vi "HEWH Panel Collect Data for Specific Time.vi"(8 "error in (no error)":errorcluster) -> (0 "error out":errorcluster, 1 "Back Button":bool, 2 "Elapsed Time Output":T2 format="%<%H:%M:%S>t", 3 "Continuous Data Collection Output":bool)   [LabVIEW 2019]
uses:
  Utility/Custom Pallet Controls/Custom Pallet Forward.ctl
  Utility/Custom Pallet Controls/Custom Pallet Timer.ctl
  Utility/Custom Pallet Controls/Custom Pallet Reverse.ctl
panel:
  in  "Back Button":T1
  out "Description":string="Data Collection Setup"
  in  "Elapsed Time":T2 format="%<%H:%M:%S>t"
  in  "Specific Time":bool
  in  "Continuous Data Collection":bool
  in  "File Setup OK":T3
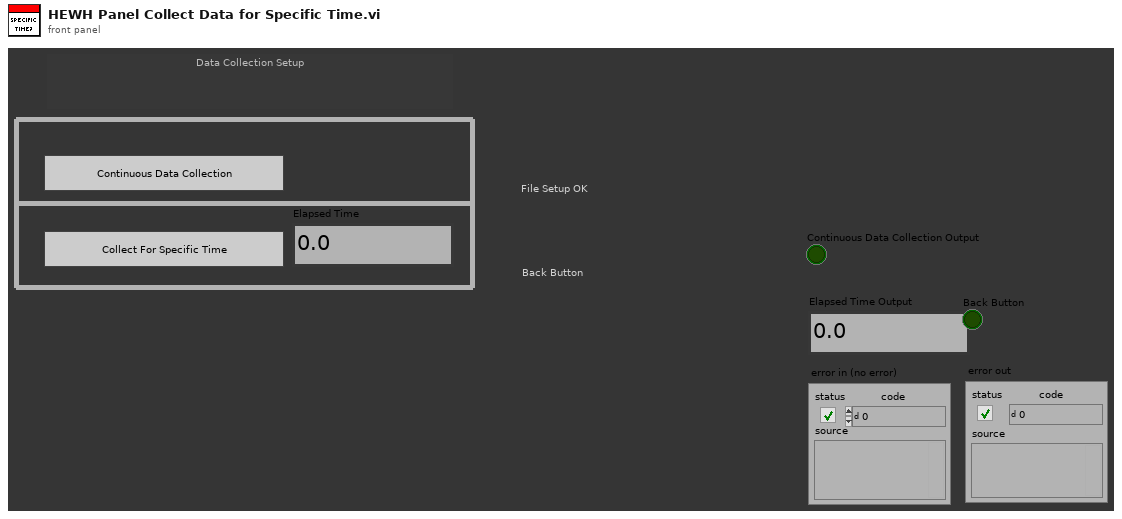
[diagram p1: front panel]
types:
  T1 = typedef "Custom Pallet Reverse.ctl" = bool
  T2 = typedef "Custom Pallet Timer.ctl" = dbl
  T3 = typedef "Custom Pallet Forward.ctl" = bool
  T4 = enum32{"invalid app kind", "Development System", "Run Time System", "Student Edition", "Embedded LabVIEW", "Evaluation", "Custom"}
  T5 = enum32{"Invalid", "Standard", "Closed", "Hidden", "Minimized", "Maximized"}
  T6 = cluster{"Core":cluster{"Current VI Reference":refnum<vi>, "Close Panel on Exit?":bool}, "Elapsed Time":T2, "Continuous Data Collection":bool}
  T7 = cluster{"Current VI Reference":refnum<vi>, "Close Panel on Exit?":bool}
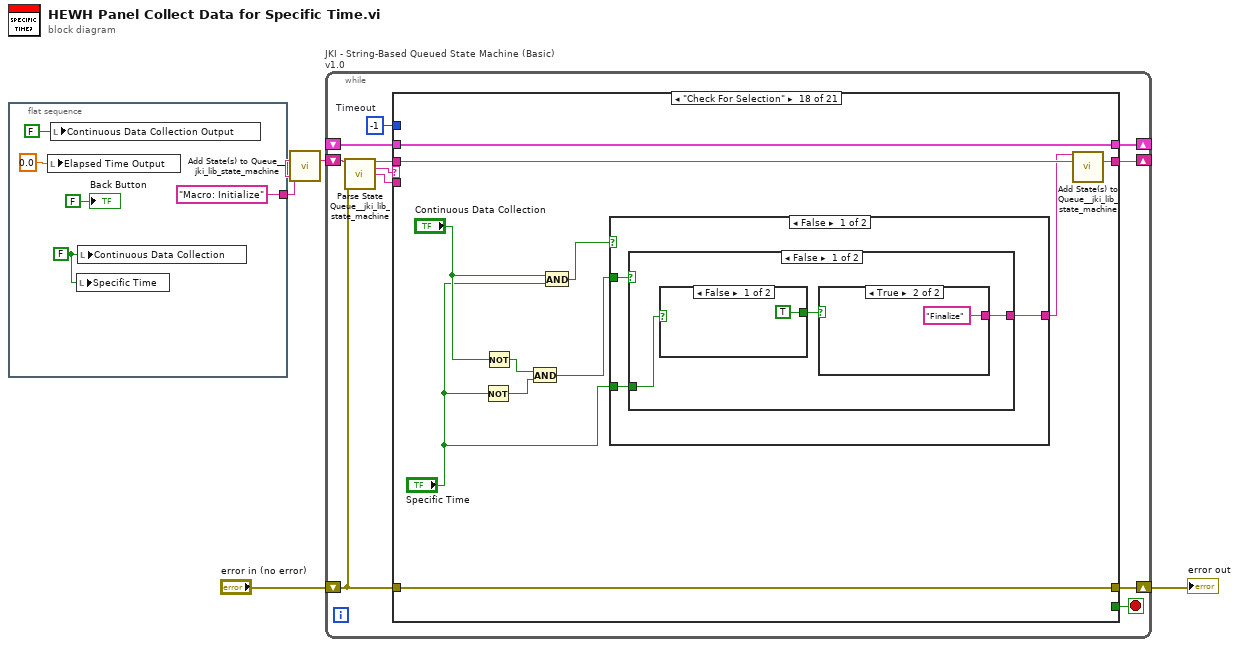
[diagram p0: block diagram]
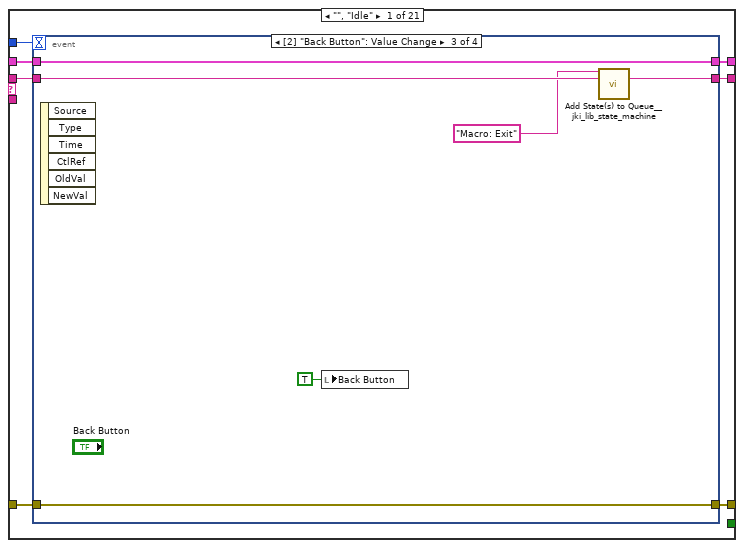
[diagram p2: hidden frame]
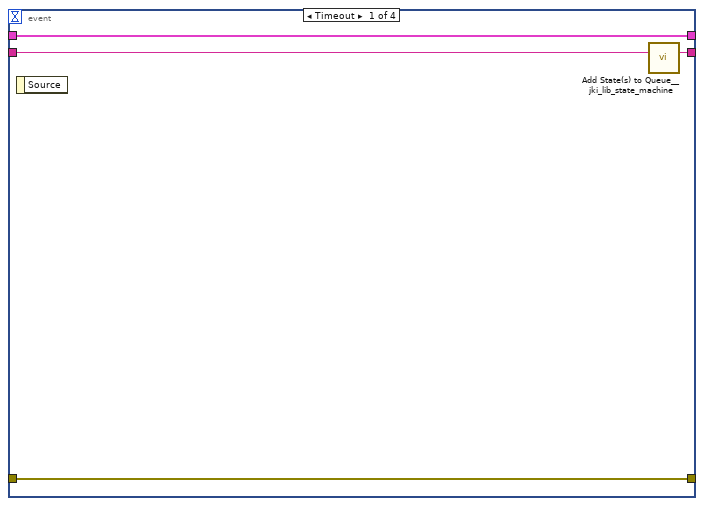
[diagram p3: hidden frame]
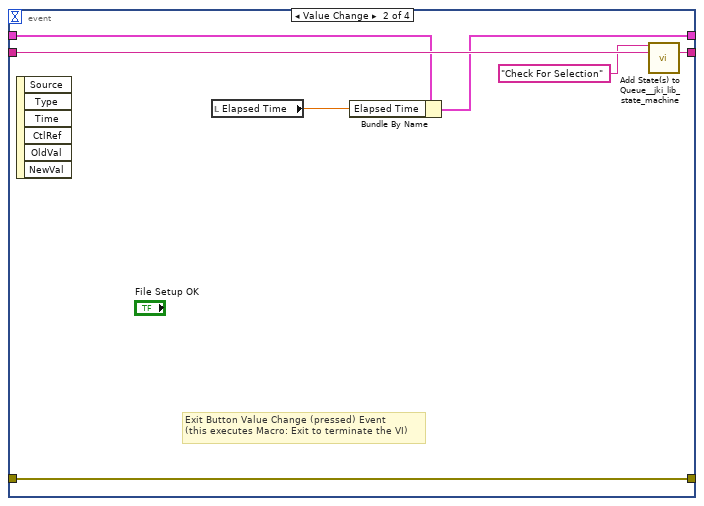
[diagram p4: hidden frame]
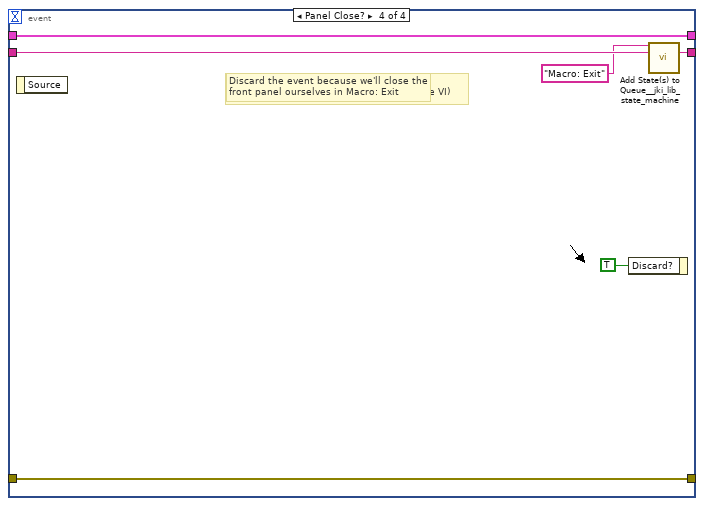
[diagram p5: hidden frame]
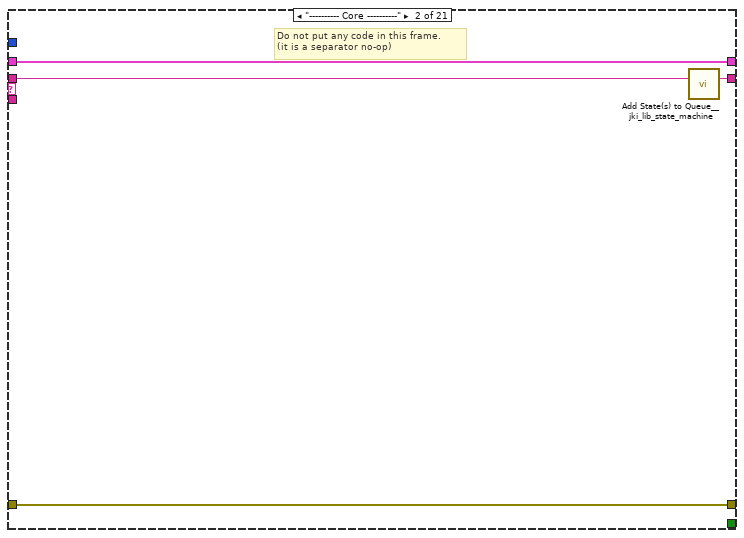
[diagram p6: hidden frame]
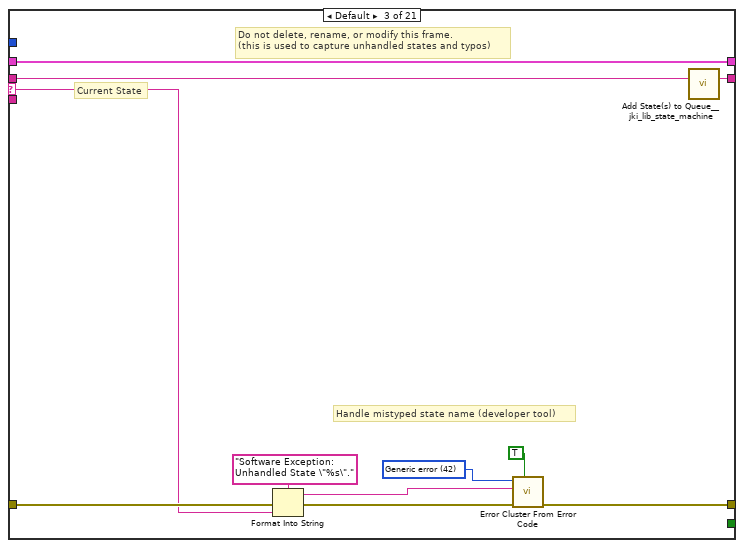
[diagram p7: hidden frame]
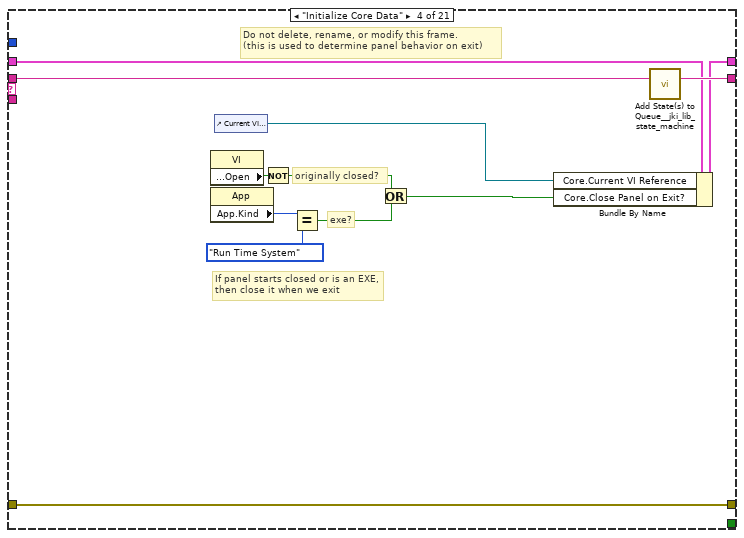
[diagram p8: hidden frame]
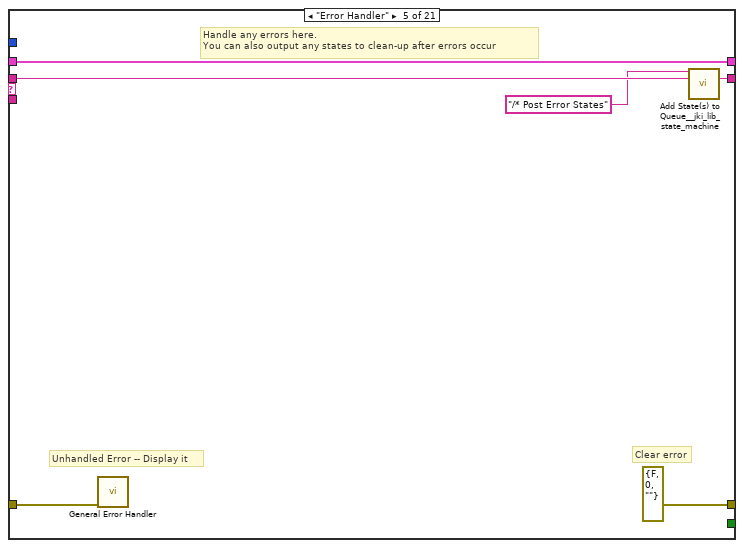
[diagram p9: hidden frame]
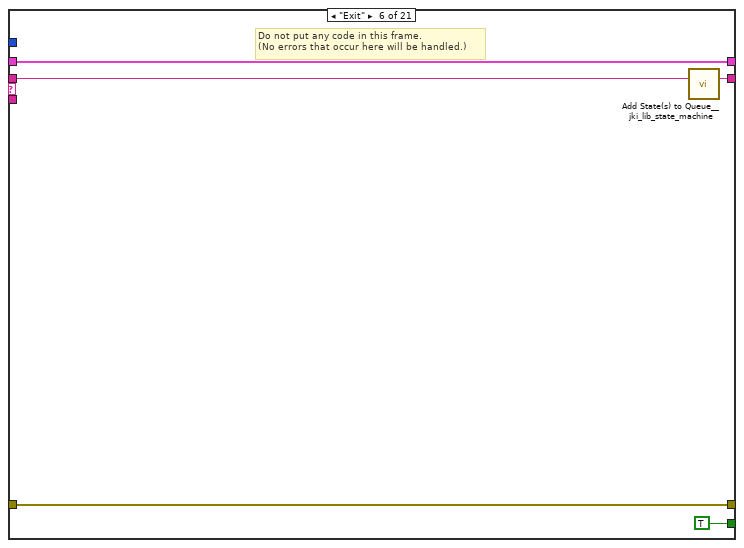
[diagram p10: hidden frame]
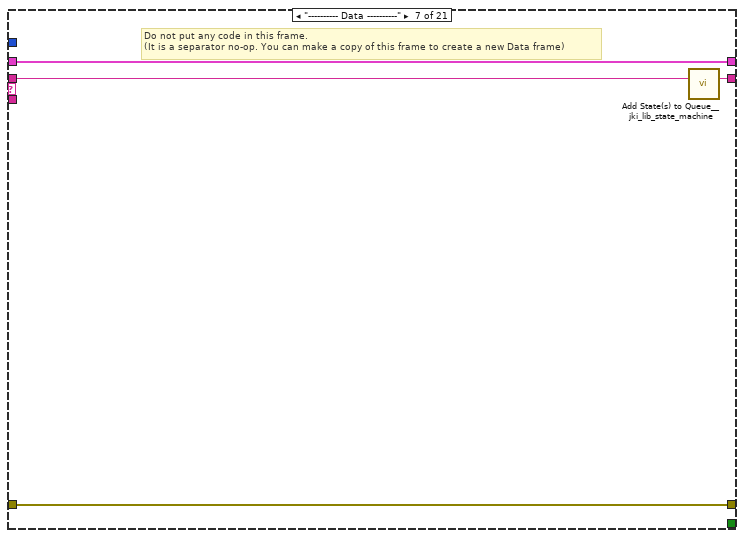
[diagram p11: hidden frame]
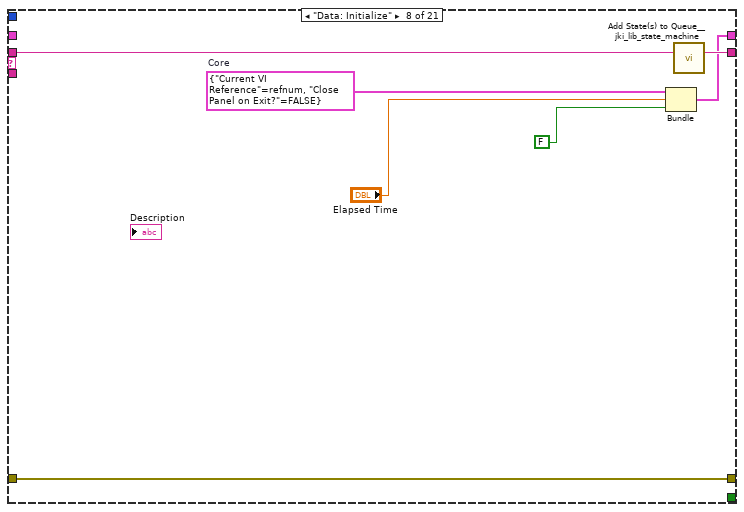
[diagram p12: hidden frame]
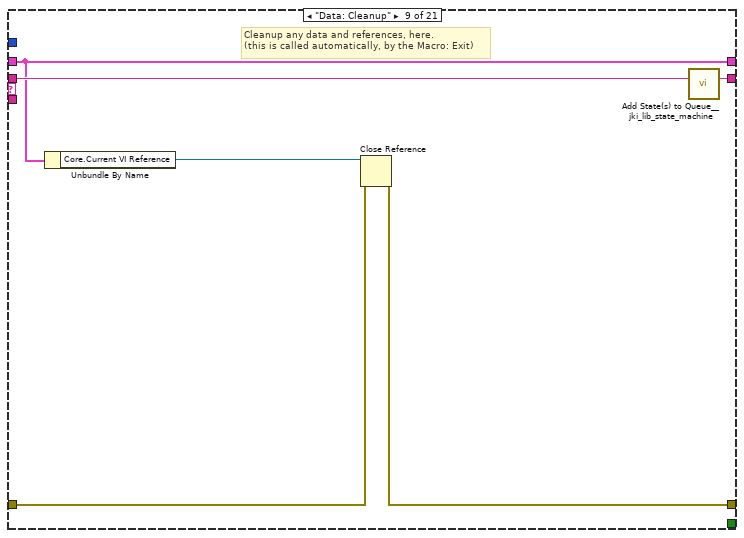
[diagram p13: hidden frame]
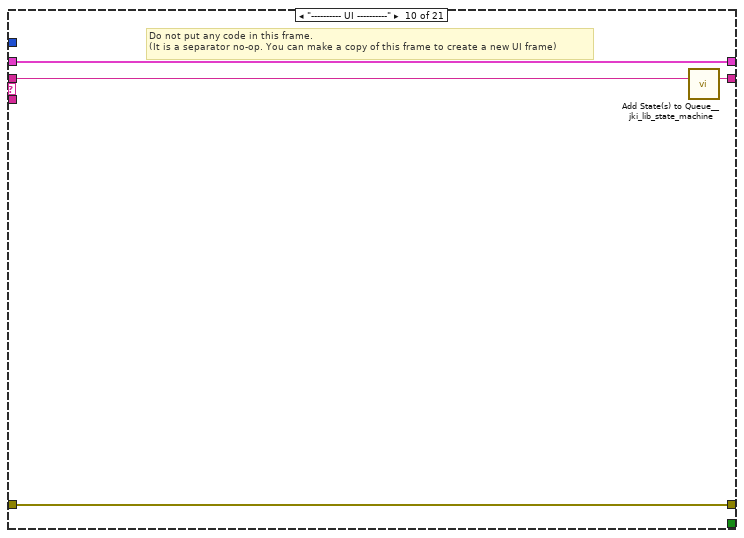
[diagram p14: hidden frame]
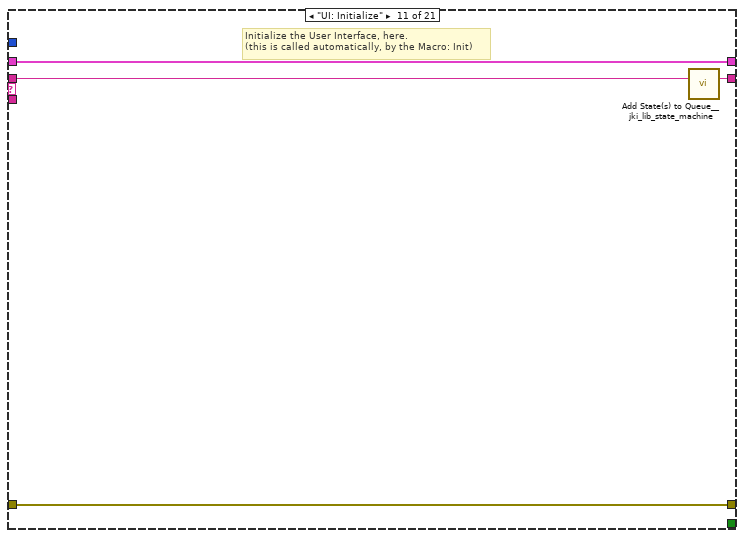
[diagram p15: hidden frame]
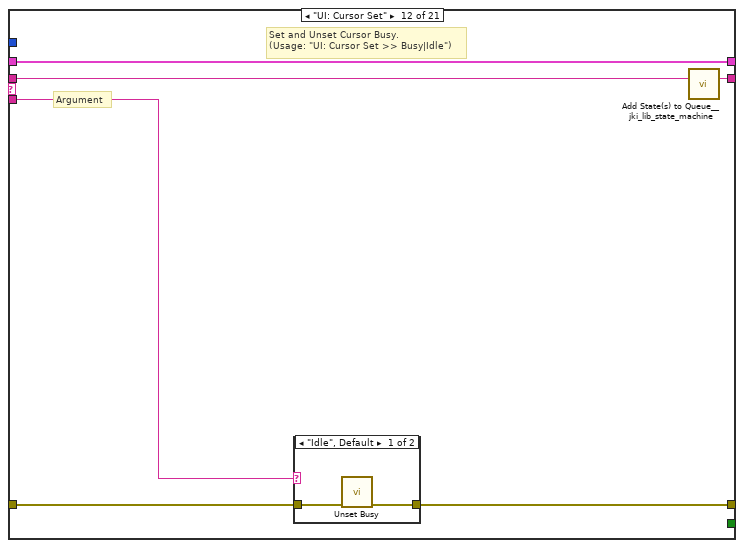
[diagram p16: hidden frame]
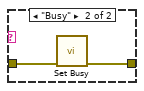
[diagram p17: hidden frame]
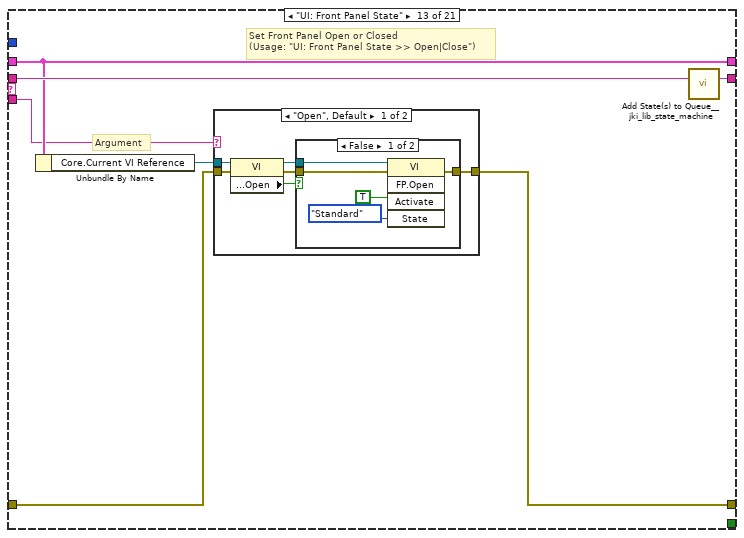
[diagram p18: hidden frame]
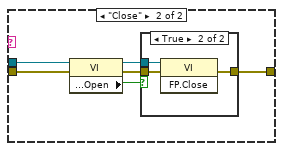
[diagram p20: hidden frame]
diagram:
  n1 = flat-sequence {
    tunnel: ["Macro: Initialize"] -> w3
    frame #0 {
      w5 = FALSE ("Continuous Data Collection")
      n2 = local write "Elapsed Time Output"(T2 0.0 ("Elapsed Time Output")) -> ()
      n3 = local write "Continuous Data Collection Output"(FALSE ("Continuous Data Collection Output")) -> ()
      n4 = local write "Specific Time"(w5) -> ()
      n5 = local write "Continuous Data Collection"(w5) -> ()
      "Back Button" <- FALSE ("Back Button")
    }
  }
  n6 = call <vilib>:"Add State(s) to Queue__jki_lib_state_machine.vi"("State(s) in (\"\")"=w3) -> ("States Out"=w4:string)  [unwired: 14 in]
  n7 = while "JKI - String-Based Queued State Machine (Basic) v1.0" {
    shift-right: [w13] -> _
    shift-left: _ -> [w12]
    shift-right: [w16] -> w2
    shift-left: "error in (no error)" -> [w10]
    shift-right: [w15] -> _
    shift-left: w4 -> [w17]
    stop <- w14 stop-if-true
    w11 = -1  # Timeout
    n8 = call <vilib>:"Parse State Queue__jki_lib_state_machine.vi"("State Queue"=w17, "Error In (no error)"=w10) -> ("Remaining States"=w19:string, "Current State"=w20:string, "Arguments"=w18:string)  [unwired: 11 in]
    n9 = case shown="\"Check For Selection\"" w20 {
      selector: w20 -> [_ _ w55 _ _ _ _ _ _ _ _ _ _ _ _ _ _ _ _ _ _]
      tunnel: w19 -> [w27 w54 w59 w77 w83 w88 w92 w99 w105 w109 w113 w119 w130 w156 w161 w171 w175 w186 w209 w221 w228]
      tunnel: w18 -> [_ _ _ _ _ _ _ _ _ _ _ w114 w124 _ _ _ _ _ _ _ _]
      tunnel: w12 -> [w25 w51 w57 w68 w80 w86 w89 _ w100 w106 w111 w117 w126 w153 w158 w168 w172 w183 w205 w218 w225]
      tunnel: [w24 w52 w61 w74 errorcluster {"status"=FALSE, "code"=0, "source"=""} ("error out") w85 w90 w96 w101 w107 w110 w115 w127 w154 w159 w169 w173 w184 w207 w219 w226] -> w16
      tunnel: w10 -> [w23 w52 w60 w74 w79 w85 w90 w96 w102 w107 w110 w116 w128 w154 w159 w169 w173 w184 w207 w219 w226]
      tunnel: [w26 w53 w58 w76 w82 w87 w91 w98 w104 w108 w112 w118 w129 w155 w160 w170 w174 w185 w208 w220 w227] -> w15
      tunnel: [_ _ _ _ _ TRUE _ _ _ _ _ _ _ _ _ _ _ _ _ _ _] -> w14
      tunnel: [w22 w51 w57 w75 w80 w86 w89 w97 w100 w106 w111 w117 w126 w153 w158 w168 w172 w183 w204 w218 w225] -> w13
      tunnel: w11 -> [w21 _ _ _ _ _ _ _ _ _ _ _ _ _ _ _ _ _ _ _ _]
      frame "", "Idle" {
        n10 = event shown="[2] \"Back Button\": Value Change" {
          selector: _ -> [_ _ _ _]
          dyn-events: _ -> [_ _ _ _]
          timeout: w21 -> [_ _ _ _]
          tunnel: w27 -> [w31 w38 w41 w50]
          tunnel: [w30 w37 w40 w49] -> w26
          tunnel: w25 -> [w28 w34 w43 w47]
          tunnel: [w29 w36 w44 w48] -> w24
          tunnel: w23 -> [w29 w36 w44 w48]
          tunnel: [w28 w33 w43 w47] -> w22
          event Timeout {
            n11 = event-data() -> ()  [unwired: 1 in, 1 out]
            n12 = call <vilib>:"Add State(s) to Queue__jki_lib_state_machine.vi"("State(s) in (\"\")"=w31) -> ("States Out"=w30:string)  [unwired: 14 in]
          }
          event Value Change {
            # "Exit Button Value Change (pressed) Event\n(this executes Macro: Exit to terminate the VI)"
            n13 = event-data() -> ()  [unwired: 1 in, 6 out]
            n14 = local read "Elapsed Time"() -> (w32:T2)
            n15 = Bundle By Name(cluster=w34, "Elapsed Time"=w32) -> (w33:T6)
            n16 = call <vilib>:"Add State(s) to Queue__jki_lib_state_machine.vi"("State(s) in Front (\"\")"="Check For Selection", "State(s) in (\"\")"=w38) -> ("States Out"=w37:string)  [unwired: 13 in]
          }
          event Value Change {
            n17 = event-data() -> ()  [unwired: 1 in, 6 out]
            n18 = local write "Back Button"(TRUE ("Back Button")) -> ()
            n19 = call <vilib>:"Add State(s) to Queue__jki_lib_state_machine.vi"("State(s) in Front (\"\")"="Macro: Exit" ("State(s) in Front (\"\")"), "State(s) in (\"\")"=w41) -> ("States Out"=w40:string)  [unwired: 13 in]
          }
          event Panel Close? {
            # "Discard the event because we'll close the front panel ourselves in Macro: Exit"
            # "Close Panel button (pressed) Event\n(this executes Macro: Exit to terminate the VI)"
            n20 = event-data() -> ()  [unwired: 1 in, 1 out]
            n21 = event-data("Discard?"=TRUE) -> ()  [unwired: 1 in, 1 out]
            n22 = call <vilib>:"Add State(s) to Queue__jki_lib_state_machine.vi"("State(s) in Front (\"\")"="Macro: Exit", "State(s) in (\"\")"=w50) -> ("States Out"=w49:string)  [unwired: 13 in]
          }
        }
      }
      frame "---------- Core ----------" {
        # "Do not put any code in this frame.\n(it is a separator no-op)"
        n23 = call <vilib>:"Add State(s) to Queue__jki_lib_state_machine.vi"("State(s) in (\"\")"=w54) -> ("States Out"=w53:string)  [unwired: 14 in]
      }
      frame Default {
        w64 = 42 items=["No error", "Argument error", "Memory is full", "Out of zone", "End of file", "File already open", "Generic file I/O error", "File not found", "File permission error", "Disk is full", "Duplicate path", "Too many files open", "System feature not enabled", "Resource file not found", "Cannot add resource", "Resource not found", "Image not found", "Image memory error", "Pen does not exist", "Config type invalid", "Config token not found", "Config parse error", "Config memory error", "Bad external code format", "Bad external code offset", "External code not present", "Null window", "Destroy window error", "Null menu", "Print aborted", "Bad print record", "Print driver error", "Windows error during printing", "Memory error during printing", "Print dialog error", "Generic print error", "Invalid device refnum", "Device not found", "Device parameter error", "Device unit error", "Cannot open device", "Device call aborted", "Generic error", "Cancelled by user", "Object ID too low", "Object ID too high", "Object not in heap", "Unknown heap", "Unknown object (invalid DefProc)", "Unknown object (DefProc not in table)", "Message out of range", "Invalid (null) method", "Unknown message", "Manager call not supported", "Bad address", "Network operation in progress", "Network operation timed out", "Connection is busy", "Network attribute not supported", "Network error", "Address in use", "System out of memory", "Connection aborted", "Connection refused", "Not connected", "Already connected", "Connection closed", "Initialization error (interapplication manager)", "Bad occurrence", "Wait on unbound occurrence handler", "Occurrence queue overflow", "Datalog type conflict", "Unused", "Unrecognized type (interapplication manager)", "Memory corrupt", "Failed to make temporary DLL", "Old CIN version", "Drag socket not found", "Failed to load drop-object", "Failed to register OLE object", "Failed to release OLE object", "Format specifier type mismatch", "Unknown format specifier", "Too few format specifiers", "Too many format specifiers", "Scan failed", "Newer CIN version", "Error converting to variant", "Runtime menu error", "Password tampered", "Variant attribute not found", "Incompatible variant data type", "Event data is not available", "Event Store is not present", "Occurrence is not found", "Event Queue is not created", "Event info is not available", "Refnum passed is NULL", "Error retrieving Class GUID", "Error retrieving CoClass GUID", "Error retrieving TypeLib GUID.", "Bad built application magic bytes.", "Specific driver is different from the specific driver associated with the Logical Name.", "There is no session opened to the class driver.", "Max Error", "MAX - Error with config objects", "MAX - Error loading configuration", "MAX - Group not supported"]
        # "Current State"
        # "Do not delete, rename, or modify this frame.\n(this is used to capture unhandled states and typos)"
        # "Handle mistyped state name (developer tool)"
        n24 = Format Into String(format string="Software Exception: Unhandled State \"%s\"." ("message"), error in=w60, w55) -> (resulting string=w63:string, error out=w62:errorcluster)  [unwired: 1 in]
        n25 = call <vilib>:"Error Cluster From Error Code.vi"("show call chain? (False)"=TRUE, "error in (no error)"=w62, "error message (\"\")"=w63, "error code (0)"=w64) -> ("error out"=w61:errorcluster)  [unwired: 5 in]
        n26 = call <vilib>:"Add State(s) to Queue__jki_lib_state_machine.vi"("State(s) in (\"\")"=w59) -> ("States Out"=w58:string)  [unwired: 14 in]
      }
      frame "Initialize Core Data" {
        # "Do not delete, rename, or modify this frame.\n(this is used to determine panel behavior on exit)"
        # "originally closed?"
        # "exe?"
        # "If panel starts closed or is an EXE, then close it when we exit"
        n27 = property class="VI"() -> ("Front Panel.Open"=w73:bool)  [unwired: 2 in, 2 out]
        n28 = property class="App"() -> ("App.Kind"=w72:T4)  [unwired: 2 in, 2 out]
        n29 = control-ref of="Current VI Reference"() -> (w66:refnum<vi>)
        n30 = Not(x=w73) -> (.not. x?=w70:bool)
        n31 = Equal?(x=w72, y=T4."Run Time System" ("Application:Kind")) -> (x = y?=w69:bool)
        n32 = Or(x=w70, y=w69) -> (x .or. y?=w67:bool)
        n33 = Bundle By Name(cluster=w68, "Core.Current VI Reference"=w66, "Core.Close Panel on Exit?"=w67) -> (w75:T6)
        n34 = call <vilib>:"Add State(s) to Queue__jki_lib_state_machine.vi"("State(s) in (\"\")"=w77) -> ("States Out"=w76:string)  [unwired: 14 in]
      }
      frame "Error Handler" {
        # "Unhandled Error -- Display it"
        # "Handle any errors here.\nYou can also output any states to clean-up after errors occur"
        # "Clear error"
        n35 = call <vilib>:"General Error Handler.vi"("error in (no error)"=w79) -> ()  [unwired: 10 in, 5 out]
        n36 = call <vilib>:"Add State(s) to Queue__jki_lib_state_machine.vi"("State(s) in Front (\"\")"="/* Post Error States", "State(s) in (\"\")"=w83) -> ("States Out"=w82:string)  [unwired: 13 in]
      }
      frame "Exit" {
        # "Do not put any code in this frame.\n(No errors that occur here will be handled.)"
        n37 = call <vilib>:"Add State(s) to Queue__jki_lib_state_machine.vi"("State(s) in (\"\")"=w88) -> ("States Out"=w87:string)  [unwired: 14 in]
      }
      frame "---------- Data ----------" {
        # "Do not put any code in this frame.\n(It is a separator no-op. You can make a copy of this frame to create a new Data frame)"
        n38 = call <vilib>:"Add State(s) to Queue__jki_lib_state_machine.vi"("State(s) in (\"\")"=w92) -> ("States Out"=w91:string)  [unwired: 14 in]
      }
      frame "Data: Initialize" {
        w95 = T7 {"Current VI Reference"=refnum, "Close Panel on Exit?"=FALSE}  # Core
        n39 = Bundle("Core"=w95, "Elapsed Time"="Elapsed Time", "Continuous Data Collection"=FALSE) -> (w97:T6)  [unwired: 1 in]
        n40 = call <vilib>:"Add State(s) to Queue__jki_lib_state_machine.vi"("State(s) in (\"\")"=w99) -> ("States Out"=w98:string)  [unwired: 14 in]
      }
      frame "Data: Cleanup" {
        # "Cleanup any data and references, here.\n(this is called automatically, by the Macro: Exit)"
        n41 = Unbundle By Name(w100) -> ("Core.Current VI Reference"=w103:refnum<vi>)
        n42 = Close Reference(reference=w103, error in (no error)=w102) -> (error out=w101:errorcluster)
        n43 = call <vilib>:"Add State(s) to Queue__jki_lib_state_machine.vi"("State(s) in (\"\")"=w105) -> ("States Out"=w104:string)  [unwired: 14 in]
      }
      frame "---------- UI ----------" {
        # "Do not put any code in this frame.\n(It is a separator no-op. You can make a copy of this frame to create a new UI frame)"
        n44 = call <vilib>:"Add State(s) to Queue__jki_lib_state_machine.vi"("State(s) in (\"\")"=w109) -> ("States Out"=w108:string)  [unwired: 14 in]
      }
      frame "UI: Initialize" {
        # "Initialize the User Interface, here.\n(this is called automatically, by the Macro: Init)"
        n45 = call <vilib>:"Add State(s) to Queue__jki_lib_state_machine.vi"("State(s) in (\"\")"=w113) -> ("States Out"=w112:string)  [unwired: 14 in]
      }
      frame "UI: Cursor Set" {
        # "Argument"
        # "Set and Unset Cursor Busy.\n(Usage: \"UI: Cursor Set >> Busy|Idle\")"
        n46 = case shown="\"Idle\", Default" w114 {
          tunnel: w116 -> [w121 w123]
          tunnel: [w120 w122] -> w115
          frame "Idle", Default {
            n47 = call <vilib>:"Unset Busy.vi"("error in (no error)"=w121) -> ("error out"=w120:errorcluster)  [unwired: 10 in]
          }
          frame "Busy" {
            n48 = call <vilib>:"Set Busy.vi"("error in (no error)"=w123) -> ("error out"=w122:errorcluster)  [unwired: 9 in, 1 out]
          }
        }
        n49 = call <vilib>:"Add State(s) to Queue__jki_lib_state_machine.vi"("State(s) in (\"\")"=w119) -> ("States Out"=w118:string)  [unwired: 14 in]
      }
      frame "UI: Front Panel State" {
        # "Argument"
        # "Set Front Panel Open or Closed\n(Usage: \"UI: Front Panel State >> Open|Close\")"
        n50 = Unbundle By Name(w126) -> ("Core.Current VI Reference"=w125:refnum<vi>)
        n51 = case shown="\"Open\", Default" w124 {
          tunnel: w128 -> [w134 w147]
          tunnel: [w136 w148] -> w127
          tunnel: w125 -> [w135 w145]
          frame "Open", Default {
            n52 = property class="VI"(reference=w135, error in=w134) -> (reference out=w132:refnum<vi>, error out=w133:errorcluster, "Front Panel.Open"=w131:bool)
            n53 = case shown="False" w131 {
              tunnel: [w139 w142] -> w136
              tunnel: w133 -> [w138 w142]
              tunnel: w132 -> [w137 _]
              frame False {
                n54 = invoke class="VI" method="FP.Open"(reference=w137, error in=w138, "Activate"=TRUE, "State"=T5."Standard") -> (error out=w139:errorcluster)  [unwired: 1 in, 4 out]
              }
              frame True {
              }
            }
          }
          frame "Close" {
            n55 = property class="VI"(reference=w145, error in=w147) -> (reference out=w144:refnum<vi>, error out=w146:errorcluster, "Front Panel.Open"=w143:bool)
            n56 = case shown="True" w143 {
              tunnel: [w149 w152] -> w148
              tunnel: w146 -> [w149 w151]
              tunnel: w144 -> [_ w150]
              frame False {
              }
              frame True {
                n57 = invoke class="VI" method="FP.Close"(reference=w150, error in=w151) -> (error out=w152:errorcluster)  [unwired: 1 in, 2 out]
              }
            }
          }
        }
        n58 = call <vilib>:"Add State(s) to Queue__jki_lib_state_machine.vi"("State(s) in (\"\")"=w130) -> ("States Out"=w129:string)  [unwired: 14 in]
      }
      frame "---------- Macro ----------" {
        # "Do not put any code in this frame.\n(It is a separator no-op. You can make a copy of this frame to create a new Macro frame)"
        n59 = call <vilib>:"Add State(s) to Queue__jki_lib_state_machine.vi"("State(s) in (\"\")"=w156) -> ("States Out"=w155:string)  [unwired: 14 in]
      }
      frame "Macro: Initialize" {
        w157 = "Data: Initialize\nInitialize Core Data\nUI: Initialize\nUI: Front Panel State >> Open"  # Data: Initialize Initialize Core Data UI: Initialize UI: Front Panel State >> Open
        # "Initialization Macro\n(This is called once, when the VI starts)"
        n60 = call <vilib>:"Add State(s) to Queue__jki_lib_state_machine.vi"("State(s) in Front (\"\")"=w157, "State(s) in (\"\")"=w161) -> ("States Out"=w160:string)  [unwired: 13 in]
      }
      frame "Macro: Exit" {
        # "Exit Macro\n(This is called once, when the VI exits)"
        n61 = Unbundle By Name(w168) -> ("Core.Close Panel on Exit?"=w167:bool)
        n62 = Select(t="UI: Front Panel State >> Close", s=w167, f="") -> (s? t:f=w164:string)
        n63 = call <vilib>:"Add State(s) to Queue__jki_lib_state_machine.vi"("State(s) in (\"\")"=w164, "State(s) at Back (\"\")"="Data: Cleanup\nExit") -> ("States Out"=w162:string)  [unwired: 13 in]
        n64 = call <vilib>:"Add State(s) to Queue__jki_lib_state_machine.vi"("State(s) in Front (\"\")"=w162, "State(s) in (\"\")"=w171) -> ("States Out"=w170:string)  [unwired: 13 in]
      }
      frame "---------- New Category ----------" {
        # "Template Separator\n(You can make a copy of, or modify, this frame)"
        n65 = call <vilib>:"Add State(s) to Queue__jki_lib_state_machine.vi"("State(s) in (\"\")"=w175) -> ("States Out"=w174:string)  [unwired: 14 in]
      }
      frame "Check For Selection" {
        n66 = Not(x="Specific Time") -> (.not. x?=w178:bool)
        n67 = Not(x="Continuous Data Collection") -> (.not. x?=w179:bool)
        n68 = And(x=w179, y=w178) -> (x .and. y?=w177:bool)
        n69 = And(x="Continuous Data Collection", y="Specific Time") -> (x .and. y?=w182:bool)
        n70 = case shown="False" w182 {
          tunnel: [w188 ""] -> w181
          tunnel: w177 -> [w189 _]
          tunnel: "Specific Time" -> [w187 _]
          frame False {
            n71 = case shown="False" w189 {
              tunnel: [w192 ""] -> w188
              tunnel: w187 -> [w190 _]
              frame False {
                n72 = case shown="False" w190 {
                  tunnel: [TRUE w194] -> w191
                  frame False {
                  }
                  frame True {
                    n73 = local read "Elapsed Time"() -> (w195:T2)
                    n74 = Greater Than 0?(x=w195) -> (x > 0?=w194:bool)
                  }
                }
                n75 = case shown="True" w191 {
                  tunnel: ["" "Finalize"] -> w192
                  frame False {
                    n76 = One Button Dialog(message="Enter A Time") -> ()  [unwired: 1 in, 1 out]
                  }
                  frame True {
                  }
                }
              }
              frame True {
                n77 = One Button Dialog(message="Select An Option") -> ()  [unwired: 1 in, 1 out]
              }
            }
          }
          frame True {
            n78 = One Button Dialog(message="Select Only One Option") -> ()  [unwired: 1 in, 1 out]
          }
        }
        n79 = call <vilib>:"Add State(s) to Queue__jki_lib_state_machine.vi"("State(s) in Front (\"\")"=w181, "State(s) in (\"\")"=w186) -> ("States Out"=w185:string)  [unwired: 13 in]
      }
      frame "Finalize" {
        n80 = local read "Continuous Data Collection"() -> (w206:bool)
        n81 = case shown="True" w206 {
          tunnel: w205 -> [w210 w215]
          tunnel: [w210 w214] -> w204
          tunnel: ["Specific Output" "Cont Output"] -> w203
          frame False {
          }
          frame True {
            n82 = Bundle By Name(cluster=w215, "Continuous Data Collection"=TRUE) -> (w214:T6)
          }
        }
        n83 = call <vilib>:"Add State(s) to Queue__jki_lib_state_machine.vi"("State(s) in Front (\"\")"=w203, "State(s) in (\"\")"=w209) -> ("States Out"=w208:string)  [unwired: 13 in]
      }
      frame "Cont Output" {
        n84 = Unbundle By Name(w218) -> ("Continuous Data Collection"=→"Continuous Data Collection Output":bool)
        n85 = call <vilib>:"Add State(s) to Queue__jki_lib_state_machine.vi"("State(s) in Front (\"\")"="Macro: Exit", "State(s) in (\"\")"=w221) -> ("States Out"=w220:string)  [unwired: 13 in]
      }
      frame "Specific Output" {
        n86 = Unbundle By Name(w225) -> ("Continuous Data Collection"=w224:bool, "Elapsed Time"=→"Elapsed Time Output":T2)
        n87 = local write "Continuous Data Collection Output"(w224) -> ()
        n88 = call <vilib>:"Add State(s) to Queue__jki_lib_state_machine.vi"("State(s) in Front (\"\")"="Macro: Exit", "State(s) in (\"\")"=w228) -> ("States Out"=w227:string)  [unwired: 13 in]
      }
    }
  }
  "error out" <- w2
